vi "Read_Img_File.vi"(4 "Divider":sgl=128.0 format="%#_13g", 6 "Shift":sgl=128.0 format="%#_13g", 7 "Dims(C,H,W)":T2, 8 "error in (no error)":errorcluster, 11 "Path":path) -> (0 "error out":errorcluster, 1 "Image(Orig)":T1, 2 "Image(Resampled)":T1, 3 "Image Data":sgl[][][](array[numeric]))   [LabVIEW 2020]
uses:
  <vilib>/Ngene/Deep Learning Toolkit/Toolkit/NN_Data/API/NN_Dims(C,H,W).ctl
  <vilib>/vision/Image Controls.llb/IMAQ Image.ctl
  <vilib>/vision/NI_Vision_Development_Module.lvlib
  <vilib>/Ngene/Deep Learning Toolkit/Toolkit/Deep_Learning_Toolkit_by_Ngene.lvlib
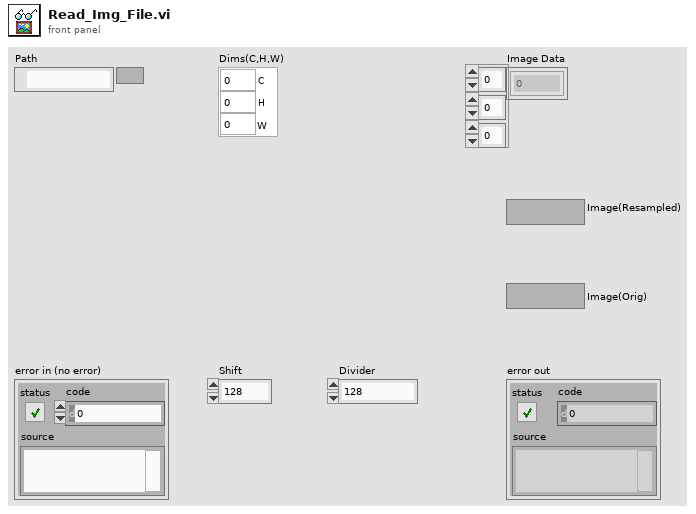
[diagram p1: front panel]
types:
  T1 = typedef "IMAQ Image.ctl" = refnum<image>
  T2 = typedef "Deep_Learning_Toolkit_by_Ngene.lvlib/NN_Dims(C,H,W).ctl" = cluster{"C":i32, "H":i32, "W":i32}
  T3 = typedef "Image Type" = u32
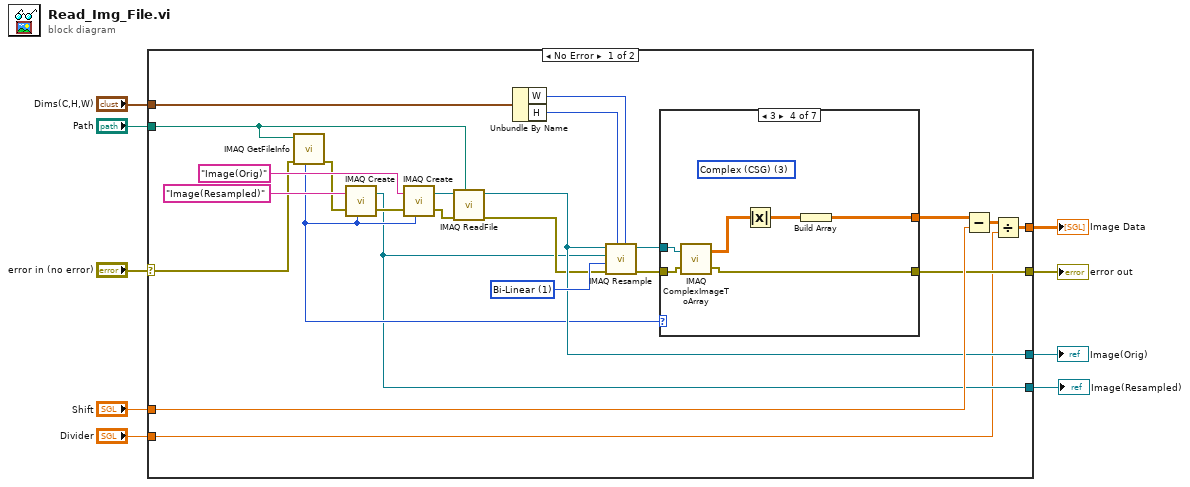
[diagram p0: block diagram]
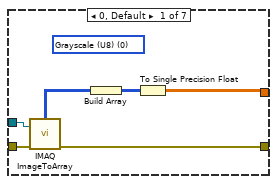
[diagram p2: hidden frame]
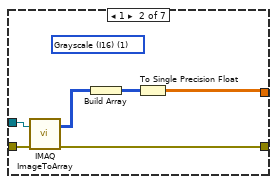
[diagram p3: hidden frame]
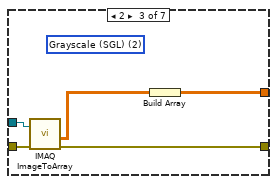
[diagram p4: hidden frame]
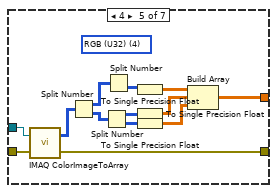
[diagram p5: hidden frame]
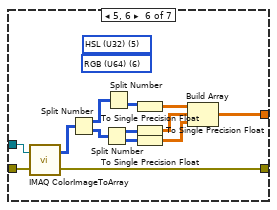
[diagram p6: hidden frame]
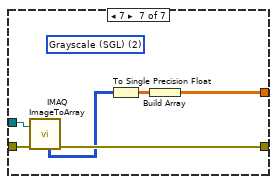
[diagram p7: hidden frame]
diagram:
  n1 = case shown="No Error" "error in (no error)" {
    selector: "error in (no error)" -> [w14 w89]
    tunnel: "Shift" -> [w31 _]
    tunnel: [w27 _] -> w8
    tunnel: [w26 w89] -> w7
    tunnel: "Dims(C,H,W)" -> [w25 _]
    tunnel: [w24 _] -> w5
    tunnel: "Path" -> [w20 _]
    tunnel: [w11 _] -> w2
    tunnel: "Divider" -> [w10 _]
    frame No Error {
      w29 = u32 1 items=["Zero Order", "Bi-Linear", "Quadratic", "Cubic Spline"] ("Interpolation Type")
      n2 = call "IMAQ GetFileInfo"("error in (no error)"=w14, "File Path"=w20) -> ("error out"=w13:errorcluster, "Image Type"=w12:T3)  [unwired: 3 in, 5 out]
      n3 = call "IMAQ Create"("Image Name"="Image(Resampled)", "Image Type"=w12, "error in (no error)"=w13) -> ("New Image"=w11:T1, "error out"=w17:errorcluster)  [unwired: 2 in]
      n4 = call "IMAQ Create"("Image Name"="Image(Orig)", "Image Type"=w12, "error in (no error)"=w17) -> ("New Image"=w19:T1, "error out"=w18:errorcluster)  [unwired: 2 in]
      n5 = call "IMAQ ReadFile"("File Path"=w20, "error in (no error)"=w18, "Image"=w19) -> ("error out"=w23:errorcluster, "Image Out"=w24:T1)  [unwired: 4 in, 3 out]
      n6 = Unbundle By Name(w25) -> ("W"=w32:i32, "H"=w33:i32)
      n7 = call "IMAQ Resample"("X Resolution"=w32, "Y Resolution"=w33, "error in (no error)"=w23, "Interpolation Type"=w29, "Image Dst"=w11, "Image Src"=w24) -> ("error out"=w22:errorcluster, "Image Dst Out"=w21:T1)  [unwired: 4 in]
      n8 = case shown="3" w12 {
        tunnel: w21 -> [w39 w45 w50 w56 w69 w82 w88]
        tunnel: w22 -> [w38 w44 w49 w55 w68 w81 w87]
        tunnel: [w36 w43 w48 w54 w66 w79 w86] -> w26
        tunnel: [w34 w41 w46 w53 w60 w73 w85] -> w28
        frame 0, Default {
          (unwired) T3 0 items=["Grayscale (U8)", "Grayscale (I16)", "Grayscale (SGL)", "Complex (CSG)", "RGB (U32)", "HSL (U32)", "RGB (U64)", "Grayscale (U16)"] ("Image Type")
          n9 = call "IMAQ ImageToArray"("error in (no error)"=w38, "Image"=w39) -> ("error out"=w36:errorcluster, "Image Pixels (U8)"=w37:u8[][])  [unwired: 2 in, 3 out]
          n10 = Build Array(w37) -> (w35:u8[][][])
          n11 = To Single Precision Float(number=w35) -> (single precision float=w34:sgl[][][])
        }
        frame 1 {
          (unwired) T3 1 items=["Grayscale (U8)", "Grayscale (I16)", "Grayscale (SGL)", "Complex (CSG)", "RGB (U32)", "HSL (U32)", "RGB (U64)", "Grayscale (U16)"] ("Image Type")
          n12 = call "IMAQ ImageToArray"("error in (no error)"=w44, "Image"=w45) -> ("error out"=w43:errorcluster, "Image Pixels (I16)"=w40:i16[][])  [unwired: 2 in, 3 out]
          n13 = Build Array(w40) -> (w42:i16[][][])
          n14 = To Single Precision Float(number=w42) -> (single precision float=w41:sgl[][][])
        }
        frame 2 {
          (unwired) T3 2 items=["Grayscale (U8)", "Grayscale (I16)", "Grayscale (SGL)", "Complex (CSG)", "RGB (U32)", "HSL (U32)", "RGB (U64)", "Grayscale (U16)"] ("Image Type")
          n15 = call "IMAQ ImageToArray"("error in (no error)"=w49, "Image"=w50) -> ("Image Pixels (Float)"=w47:sgl[][], "error out"=w48:errorcluster)  [unwired: 2 in, 3 out]
          n16 = Build Array(w47) -> (w46:sgl[][][])
        }
        frame 3 {
          (unwired) T3 3 items=["Grayscale (U8)", "Grayscale (I16)", "Grayscale (SGL)", "Complex (CSG)", "RGB (U32)", "HSL (U32)", "RGB (U64)", "Grayscale (U16)"] ("Image Type")
          n17 = call "IMAQ ComplexImageToArray"("Image"=w56, "error in (no error)"=w55) -> ("Image Pixels (Complex)"=w52:csg[][], "error out"=w54:errorcluster)  [unwired: 3 in]
          n18 = Absolute Value(x=w52) -> (abs(x)=w51:sgl[][])
          n19 = Build Array(w51) -> (w53:sgl[][][])
        }
        frame 4 {
          (unwired) T3 4 items=["Grayscale (U8)", "Grayscale (I16)", "Grayscale (SGL)", "Complex (CSG)", "RGB (U32)", "HSL (U32)", "RGB (U64)", "Grayscale (U16)"] ("Image Type")
          n20 = call "IMAQ ColorImageToArray"("Image"=w69, "error in (no error)"=w68) -> ("Image Pixels (U32)"=w67:u32[][], "error out"=w66:errorcluster)  [unwired: 2 in, 1 out]
          n21 = Split Number(x=w67) -> (hi(x)=w64:u16[][], lo(x)=w65:u16[][])
          n22 = Split Number(x=w65) -> (hi(x)=w62:u8[][], lo(x)=w61:u8[][])
          n23 = Split Number(x=w64) -> (lo(x)=w63:u8[][])  [unwired: 1 out]
          n24 = To Single Precision Float(number=w63) -> (single precision float=w59:sgl[][])
          n25 = To Single Precision Float(number=w62) -> (single precision float=w58:sgl[][])
          n26 = To Single Precision Float(number=w61) -> (single precision float=w57:sgl[][])
          n27 = Build Array(w59, w58, w57) -> (w60:sgl[][][])
        }
        frame 5, 6 {
          (unwired) T3 6 items=["Grayscale (U8)", "Grayscale (I16)", "Grayscale (SGL)", "Complex (CSG)", "RGB (U32)", "HSL (U32)", "RGB (U64)", "Grayscale (U16)"] ("Image Type")
          (unwired) T3 5 items=["Grayscale (U8)", "Grayscale (I16)", "Grayscale (SGL)", "Complex (CSG)", "RGB (U32)", "HSL (U32)", "RGB (U64)", "Grayscale (U16)"] ("Image Type")
          n28 = call "IMAQ ColorImageToArray"("Image"=w82, "error in (no error)"=w81) -> ("Image Pixels (U32)"=w80:u32[][], "error out"=w79:errorcluster)  [unwired: 2 in, 1 out]
          n29 = Split Number(x=w80) -> (hi(x)=w77:u16[][], lo(x)=w78:u16[][])
          n30 = Split Number(x=w78) -> (hi(x)=w75:u8[][], lo(x)=w74:u8[][])
          n31 = Split Number(x=w77) -> (lo(x)=w76:u8[][])  [unwired: 1 out]
          n32 = To Single Precision Float(number=w76) -> (single precision float=w72:sgl[][])
          n33 = To Single Precision Float(number=w75) -> (single precision float=w71:sgl[][])
          n34 = To Single Precision Float(number=w74) -> (single precision float=w70:sgl[][])
          n35 = Build Array(w72, w71, w70) -> (w73:sgl[][][])
        }
        frame 7 {
          (unwired) T3 2 items=["Grayscale (U8)", "Grayscale (I16)", "Grayscale (SGL)", "Complex (CSG)", "RGB (U32)", "HSL (U32)", "RGB (U64)", "Grayscale (U16)"] ("Image Type")
          n36 = call "IMAQ ImageToArray"("error in (no error)"=w87, "Image"=w88) -> ("Image Pixels (U16)"=w84:u16[][], "error out"=w86:errorcluster)  [unwired: 2 in, 3 out]
          n37 = To Single Precision Float(number=w84) -> (single precision float=w83:sgl[][])
          n38 = Build Array(w83) -> (w85:sgl[][][])
        }
      }
      n39 = Subtract(x=w28, y=w31) -> (x-y=w30:sgl[][][])
      n40 = Divide(x=w30, y=w10) -> (x/y=w27:sgl[][][])
    }
    frame Error {
    }
  }
  "Image Data" <- w8
  "error out" <- w7
  "Image(Orig)" <- w5
  "Image(Resampled)" <- w2
